vi "Configure Generator Frequency And Level.vi"(7 "Level (-30.0)":dbl=-30.0 format="%^.3e", 8 "error in (no error)":errorcluster, 9 "Frequency (1.2GHz)":dbl=1200000000.0 format="%#.9p", 10 "Instance (1)":i32=1 format="%.0g", 11 "VISA resource name":refnum<visa-resource-name>) -> (0 "error out":errorcluster, 3 "VISA resource name out":refnum<visa-resource-name>)   [LabVIEW 2020, in "Rohde&Schwarz CMXP GPRF.lvlib"]
doc: "Configures the constant-frequency generator mode.\n\nAttributes:\nRSCMXPGPRF_ATTR_GENERATOR_FREQUENCY\nRSCMXPGPRF_ATTR_GENERATOR_BASE_LEVEL\n\nRemote-control commands:\nSOURce:GPRF:GEN<i>:RFSettings:FREQuency\nSOURce:GPRF:GEN<i>:RFSettings:LEVel"
uses:
  <instrlib>/Rohde&Schwarz CMXP GPRF/Rohde&Schwarz CMXP GPRF.lvlib
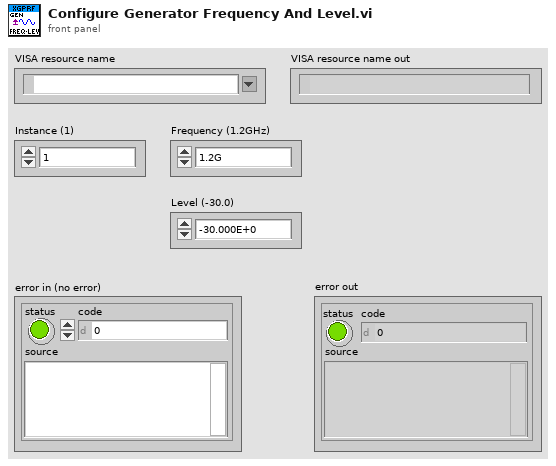
[diagram p1: front panel]
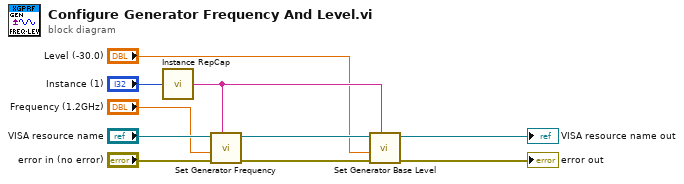
[diagram p0: block diagram]
diagram:
  n1 = call <instrlib>:"Instance RepCap.vi"("Instance in"="Instance (1)") -> ("Instance out"=w3:string)
  n2 = call "Set Generator Frequency"("Repeated Capabilities"=w3, "error in (no error)"="error in (no error)", "Generator Frequency (0.0)"="Frequency (1.2GHz)", "instrument handle"="VISA resource name") -> ("error out"=w6:errorcluster, "instrument handle out"=w7:refnum<visa-resource-name>)  [unwired: 6 in]
  n3 = call "Set Generator Base Level"("Repeated Capabilities"=w3, "error in (no error)"=w6, "Generator Base Level (0.0)"="Level (-30.0)", "instrument handle"=w7) -> ("error out"=→"error out":errorcluster, "instrument handle out"=→"VISA resource name out":refnum<visa-resource-name>)  [unwired: 6 in]
